vi "Overlay Results (Clamp).vi"(4 "Min / Max":bool, 5 "Setup":T3, 6 "Perpendicular Lines":T2(array[cluster]) {"?"."Y" format="%.2f"; "?"."X" format="%.2f"; "?"."Y" format="%.2f"; "?"."X" format="%.2f"}, 7 "ROI Descriptor":T1 {"Contours"."Type" items=["No Selection", "Point", "Line", "Rectangle", "Oval", "Polygon", "Free", "Annulus", "Unused2", "Unused3", "Broken Line", "Free Hand Line", "Rotated Rectangle"]}, 8 "Search Lines":T2(array[cluster]) {"?"."Y" format="%.2f"; "?"."X" format="%.2f"; "?"."Y" format="%.2f"; "?"."X" format="%.2f"}, 9 "All Edges Found":cluster{"X":sgl, "Y":sgl}[](array[cluster])=[{"X"=27.450102, "Y"=144.0}, {"X"=70.80146, "Y"=144.0}, {"X"=114.11963, "Y"=144.0}, {"X"=158.60345, "Y"=144.0}, {"X"=202.3678, "Y"=144.0}, {"X"=246.04292, "Y"=144.0}, {"X"=291.42203, "Y"=144.0}, {"X"=336.54822, "Y"=144.0}, {"X"=379.2348, "Y"=144.0}, {"X"=425.02194, "Y"=144.0}, {"X"=467.72144, "Y"=144.0}, {"X"=26.88918, "Y"=210.0}, {"X"=70.6191, "Y"=210.0}, {"X"=115.31038, "Y"=210.0}, {"X"=159.03351, "Y"=210.0}, {"X"=202.2118, "Y"=210.0}, {"X"=247.37573, "Y"=210.0}, {"X"=292.001, "Y"=210.0}, {"X"=336.55954, "Y"=210.0}, {"X"=379.72208, "Y"=210.0}, {"X"=424.86005, "Y"=210.0}, {"X"=468.8485, "Y"=210.0}, {"X"=26.897532, "Y"=309.0}, {"X"=70.88008, "Y"=309.0}, {"X"=114.93419, "Y"=309.0}, {"X"=159.13483, "Y"=309.0}, {"X"=203.12064, "Y"=309.0}, {"X"=247.9202, "Y"=309.0}, {"X"=291.07425, "Y"=309.0}, {"X"=335.25354, "Y"=309.0}, {"X"=378.88284, "Y"=309.0}, {"X"=424.06085, "Y"=309.0}, {"X"=469.80658, "Y"=309.0}] {"Y" format="%.2f"; "X" format="%.2f"}, 10 "Measurement Edges":cluster{"X":sgl, "Y":sgl}[](array[cluster])=[{"X"=27.450102, "Y"=144.0}, {"X"=70.80146, "Y"=144.0}, {"X"=114.11963, "Y"=144.0}, {"X"=158.60345, "Y"=144.0}, {"X"=202.3678, "Y"=144.0}, {"X"=246.04292, "Y"=144.0}, {"X"=291.42203, "Y"=144.0}, {"X"=336.54822, "Y"=144.0}, {"X"=379.2348, "Y"=144.0}, {"X"=425.02194, "Y"=144.0}, {"X"=467.72144, "Y"=144.0}, {"X"=26.88918, "Y"=210.0}, {"X"=70.6191, "Y"=210.0}, {"X"=115.31038, "Y"=210.0}, {"X"=159.03351, "Y"=210.0}, {"X"=202.2118, "Y"=210.0}, {"X"=247.37573, "Y"=210.0}, {"X"=292.001, "Y"=210.0}, {"X"=336.55954, "Y"=210.0}, {"X"=379.72208, "Y"=210.0}, {"X"=424.86005, "Y"=210.0}, {"X"=468.8485, "Y"=210.0}, {"X"=26.897532, "Y"=309.0}, {"X"=70.88008, "Y"=309.0}, {"X"=114.93419, "Y"=309.0}, {"X"=159.13483, "Y"=309.0}, {"X"=203.12064, "Y"=309.0}, {"X"=247.9202, "Y"=309.0}, {"X"=291.07425, "Y"=309.0}, {"X"=335.25354, "Y"=309.0}, {"X"=378.88284, "Y"=309.0}, {"X"=424.06085, "Y"=309.0}, {"X"=469.80658, "Y"=309.0}] {"Y" format="%.2f"; "X" format="%.2f"}, 11 "Image In":T4) -> (3 "Image Out":T4)   [LabVIEW 2020]
uses:
  IMAQ Image.ctl
panel:
  in  "Result Color":u32(colorbox)=16711680
  in  "Edge Locations Color":u32(colorbox)=16776960
  in  "Search Lines Color":u32(colorbox)=26367
  in  "Search Area Color":u32(colorbox)=65280
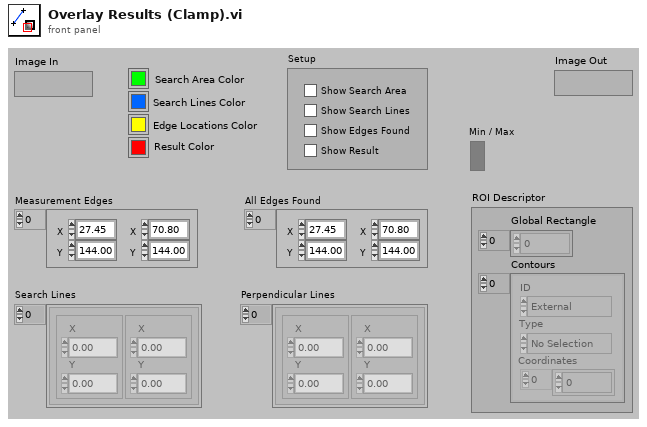
[diagram p1: front panel]
types:
  T1 = cluster{"Global Rectangle":i32[], "Contours":cluster{"ID":enum32{"External", "Internal"}, "Type":u32, "Coordinates":i32[]}[]}
  T2 = cluster{cluster{"X":sgl, "Y":sgl}, cluster{"X":sgl, "Y":sgl}}[]
  T3 = cluster{"Show Search Area":bool, "Show Search Lines":bool, "Show Edges Found":bool, "Show Result":bool}
  T4 = typedef "IMAQ Image.ctl" = refnum<image>
  T5 = cluster{"[0]":sgl, "[1]":sgl, "[2]":sgl, "[3]":sgl}
  T6 = cluster{"Perpendicular Lines[0]":cluster{cluster{"X":sgl, "Y":sgl}, cluster{"X":sgl, "Y":sgl}}, "Perpendicular Lines[1]":cluster{cluster{"X":sgl, "Y":sgl}, cluster{"X":sgl, "Y":sgl}}}
  T7 = cluster{cluster{"X":sgl, "Y":sgl}, cluster{"X":sgl, "Y":sgl}}
  T8 = cluster{cluster{"X":dbl, "Y":dbl}, cluster{"X":dbl, "Y":dbl}}
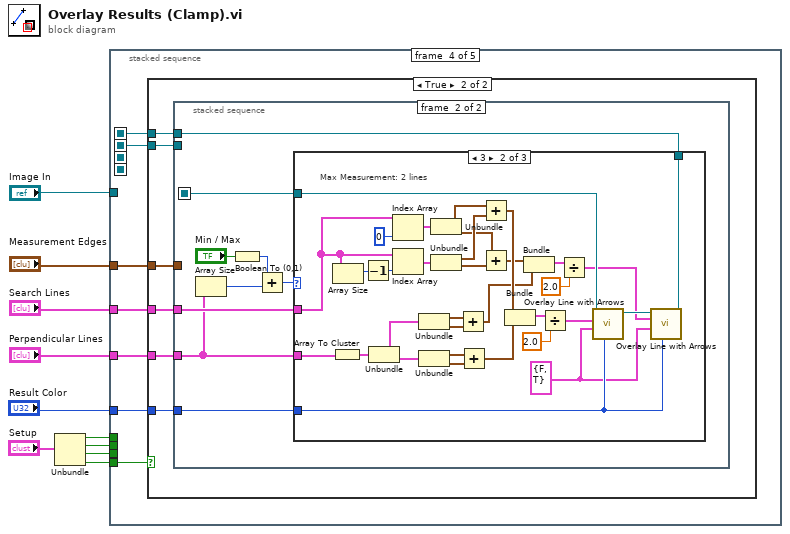
[diagram p0: block diagram]
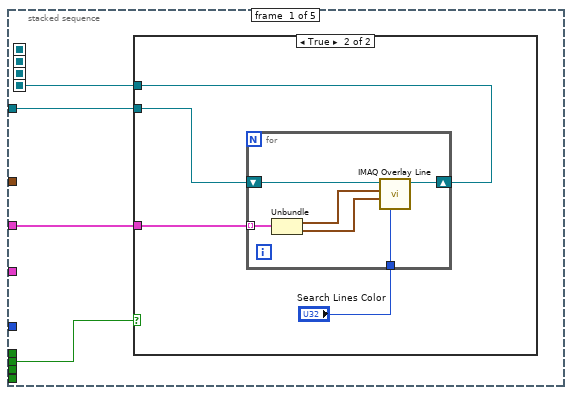
[diagram p2: hidden frame]
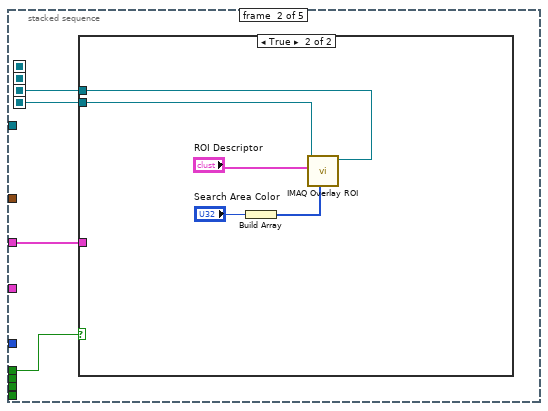
[diagram p4: hidden frame]
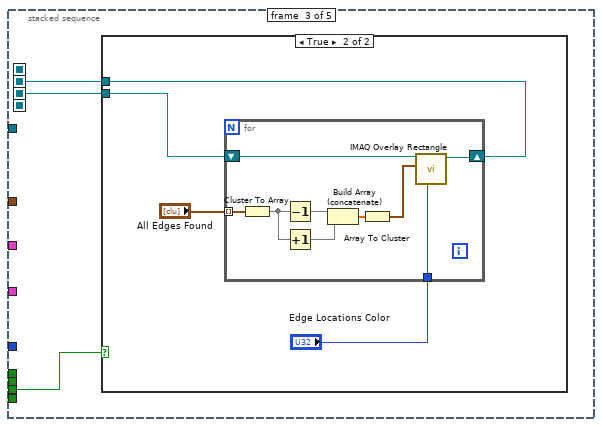
[diagram p6: hidden frame]
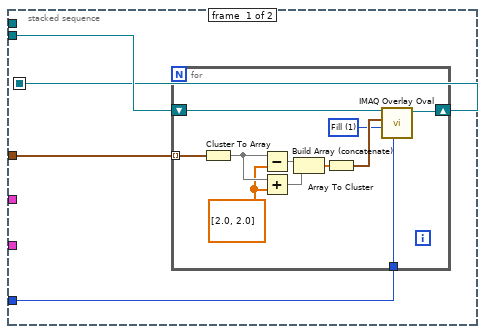
[diagram p9: hidden frame]
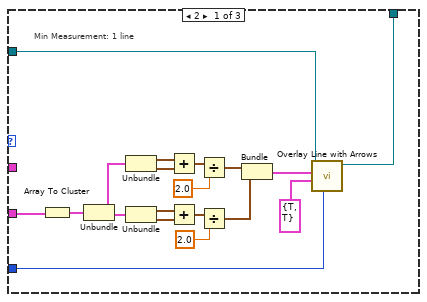
[diagram p10: hidden frame]
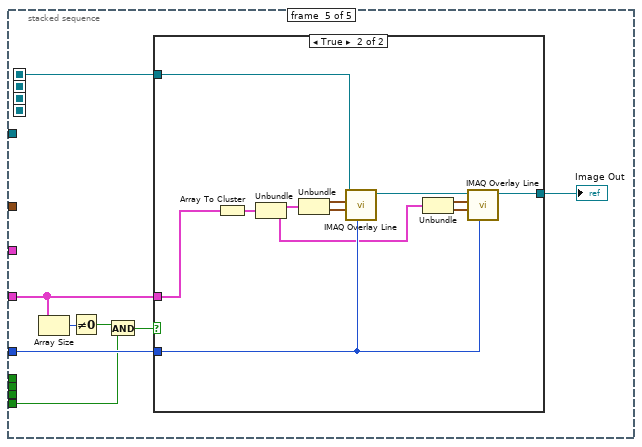
[diagram p12: hidden frame]
diagram:
  n1 = Unbundle("Setup") -> ("Show Search Area"=w4:bool, "Show Search Lines"=w5:bool, "Show Edges Found"=w3:bool, "Show Result"=w2:bool)
  n2 = stacked-sequence {
    seq-local: [_ _ w38 _ _] -> [_ _ _ w59 _]
    seq-local: [w13 _ _ _ _] -> [_ w28 _ _ _]
    seq-local: [_ w29 _ _ _] -> [_ _ w37 _ _]
    seq-local: [_ _ _ w58 _] -> [_ _ _ _ w149]
    tunnel: "Image In" -> [w14 _ _ _ _]
    tunnel: "Search Lines" -> [w12 w27 _ w53 _]
    tunnel: "Result Color" -> [_ _ _ w57 w150]
    tunnel: "Measurement Edges" -> [_ _ _ w56 _]
    tunnel: w5 -> [w11 _ _ _ _]
    tunnel: w4 -> [_ w26 _ _ _]
    tunnel: w3 -> [_ _ w36 _ _]
    tunnel: w2 -> [_ _ _ w55 w145]
    tunnel: "Perpendicular Lines" -> [_ _ _ w54 w148]
    frame #0 {
      n3 = case shown="True" w11 {
        tunnel: w14 -> [w15 w19]
        tunnel: [w15 w17] -> w13
        tunnel: w12 -> [_ w16]
        frame False {
        }
        frame True {
          n4 = for {
            shift-right: [w25] -> w17
            shift-left: w19 -> [w21]
            tunnel: "Search Lines Color" -> [w24]
            tunnel: w16 -> [w23] mode=indexing
            n5 = Unbundle(w23) -> (w20:cluster{"X":sgl, "Y":sgl}, w22:cluster{"X":sgl, "Y":sgl})
            n6 = call "IMAQ Overlay Line"("Color"=w24, "End Point"=w22, "Start Point"=w20, "Image"=w21) -> ("Image Out"=w25:T4)  [unwired: 2 in, 5 out]
          }
        }
      }
    }
    frame #1 {
      n7 = case shown="True" w26 {
        tunnel: [w30 w33] -> w29
        tunnel: w28 -> [w30 w34]
        tunnel: w27 -> [_ _]
        frame False {
        }
        frame True {
          n8 = Build Array("Search Area Color") -> (w31:u32[])
          n9 = call "IMAQ Overlay ROI"("Colors (Green)"=w31, "ROI Descriptor"="ROI Descriptor", "Image"=w34) -> ("Image Out"=w33:T4)  [unwired: 3 in, 5 out]
        }
      }
    }
    frame #2 {
      n10 = case shown="True" w36 {
        tunnel: [w39 w43] -> w38
        tunnel: w37 -> [w39 w42]
        frame False {
        }
        frame True {
          n11 = for {
            shift-right: [w51] -> w43
            shift-left: w42 -> [w52]
            tunnel: "All Edges Found" -> [w50] mode=indexing
            tunnel: "Edge Locations Color" -> [w49]
            n12 = Cluster To Array(cluster=w50) -> (array=w45:sgl[])
            n13 = Decrement(x=w45) -> (x-1=w48:sgl[])
            n14 = Increment(x=w45) -> (x+1=w44:sgl[])
            n15 = Build Array (concatenate)(w48, w44) -> (w47:sgl[])
            n16 = Array To Cluster(array=w47) -> (cluster=w46:T5)
            n17 = call "IMAQ Overlay Rectangle"("Color"=w49, "Rectangle"=w46, "Image"=w52) -> ("Image Out"=w51:T4)  [unwired: 3 in, 5 out]
          }
        }
      }
    }
    frame #3 {
      n18 = case shown="True" w55 {
        tunnel: w59 -> [w60 w66]
        tunnel: [w60 w63] -> w58
        tunnel: w57 -> [_ w65]
        tunnel: w56 -> [_ w64]
        tunnel: w54 -> [_ w62]
        tunnel: w53 -> [_ w61]
        frame False {
        }
        frame True {
          n19 = stacked-sequence {
            seq-local: [w67 _] -> [_ w89]
            tunnel: w66 -> [w70 _]
            tunnel: w65 -> [w69 w90]
            tunnel: w64 -> [w68 _]
            tunnel: [_ w88] -> w63
            tunnel: w62 -> [_ w86]
            tunnel: w61 -> [_ w87]
            frame #0 {
              n20 = for {
                shift-right: [w80] -> w67
                shift-left: w70 -> [w81]
                tunnel: w68 -> [w79] mode=indexing
                tunnel: w69 -> [w72]
                w71 = u32 1 items=["Frame", "Fill"] ("Drawing Mode (Frame)")
                w73 = sgl[] [2.0, 2.0] ("y")
                n21 = Cluster To Array(cluster=w79) -> (array=w78:sgl[])
                n22 = Subtract(x=w78, y=w73) -> (x-y=w77:sgl[])
                n23 = Add(x=w78, y=w73) -> (x+y=w76:sgl[])
                n24 = Build Array (concatenate)(w77, w76) -> (w75:sgl[])
                n25 = Array To Cluster(array=w75) -> (cluster=w74:T5)
                n26 = call "IMAQ Overlay Oval"("Color"=w72, "Drawing Mode (Frame)"=w71, "Bounding Rectangle"=w74, "Image"=w81) -> ("Image Out"=w80:T4)  [unwired: 2 in, 5 out]
              }
            }
            frame #1 {
              n27 = Array Size(array=w86) -> (size(s)=w84:i32)
              n28 = Boolean To (0,1)(Boolean="Min / Max") -> (0, 1=w83:i16)
              n29 = Add(x=w83, y=w84) -> (x+y=w82:i32)
              n30 = case shown="3" w82 {
                tunnel: w90 -> [w109 w126 _]
                tunnel: w89 -> [w108 w142 w143]
                tunnel: [w107 w124 w143] -> w88
                tunnel: w86 -> [w91 w134 _]
                tunnel: w87 -> [_ w128 _]
                frame 2 {
                  # "Min Measurement: 1 line"
                  n31 = Array To Cluster(array=w91) -> (cluster=w104:T6)
                  n32 = Unbundle(w104) -> ("Perpendicular Lines[0]"=w103:T7, "Perpendicular Lines[1]"=w94:T7)
                  n33 = Unbundle(w103) -> (w102:cluster{"X":sgl, "Y":sgl}, w101:cluster{"X":sgl, "Y":sgl})
                  n34 = Unbundle(w94) -> (w95:cluster{"X":sgl, "Y":sgl}, w96:cluster{"X":sgl, "Y":sgl})
                  n35 = Add(x=w102, y=w101) -> (x+y=w100:cluster{"X":sgl, "Y":sgl})
                  n36 = Add(x=w95, y=w96) -> (x+y=w97:cluster{"X":sgl, "Y":sgl})
                  n37 = Divide(x=w100, y=2.0) -> (x/y=w93:cluster{"X":dbl, "Y":dbl})
                  n38 = Divide(x=w97, y=2.0) -> (x/y=w92:cluster{"X":dbl, "Y":dbl})
                  n39 = Bundle(w93, w92) -> (w105:T8)  [unwired: 1 out]
                  n40 = call "Overlay Line with Arrows.vi"("Color"=w109, "Arrows"=cluster{"Start point":bool, "End point":bool} {"Start point"=TRUE, "End point"=TRUE}, "Line Coordinates"=w105, "Image In"=w108) -> ("Image Out"=w107:T4)  [unwired: 2 in, 5 out]
                }
                frame 3 {
                  w125 = cluster{"Start point":bool, "End point":bool} {"Start point"=FALSE, "End point"=TRUE} ("Arrows")
                  # "Max Measurement: 2 lines"
                  n41 = Array To Cluster(array=w134) -> (cluster=w141:T6)
                  n42 = Array Size(array=w128) -> (size(s)=w133:i32)
                  n43 = Decrement(x=w133) -> (x-1=w132:i32)
                  n44 = Unbundle(w141) -> ("Perpendicular Lines[0]"=w140:T7, "Perpendicular Lines[1]"=w135:T7)
                  n45 = Index Array(array=w128, index=0 ("Index")) -> (element=w131:T7)
                  n46 = Index Array(array=w128, index=w132) -> (element=w130:T7)
                  n47 = Unbundle(w140) -> (w139:cluster{"X":sgl, "Y":sgl}, w138:cluster{"X":sgl, "Y":sgl})
                  n48 = Unbundle(w135) -> (w136:cluster{"X":sgl, "Y":sgl}, w137:cluster{"X":sgl, "Y":sgl})
                  n49 = Unbundle(w131) -> (w123:cluster{"X":sgl, "Y":sgl}, w121:cluster{"X":sgl, "Y":sgl})
                  n50 = Unbundle(w130) -> (w122:cluster{"X":sgl, "Y":sgl}, w120:cluster{"X":sgl, "Y":sgl})
                  n51 = Add(x=w139, y=w138) -> (x+y=w117:cluster{"X":sgl, "Y":sgl})
                  n52 = Add(x=w136, y=w137) -> (x+y=w116:cluster{"X":sgl, "Y":sgl})
                  n53 = Add(x=w123, y=w122) -> (x+y=w119:cluster{"X":sgl, "Y":sgl})
                  n54 = Add(x=w121, y=w120) -> (x+y=w118:cluster{"X":sgl, "Y":sgl})
                  n55 = Bundle(w119, w116) -> (w115:T7)  [unwired: 1 out]
                  n56 = Bundle(w118, w117) -> (w113:T7)  [unwired: 1 out]
                  n57 = Divide(x=w115, y=2.0) -> (x/y=w114:T8)
                  n58 = Divide(x=w113, y=2.0) -> (x/y=w112:T8)
                  n59 = call "Overlay Line with Arrows.vi"("Color"=w126, "Arrows"=w125, "Line Coordinates"=w114, "Image In"=w142) -> ("Image Out"=w127:T4)  [unwired: 2 in, 5 out]
                  n60 = call "Overlay Line with Arrows.vi"("Color"=w126, "Arrows"=w125, "Line Coordinates"=w112, "Image In"=w127) -> ("Image Out"=w124:T4)  [unwired: 2 in, 5 out]
                }
                frame Default {
                  # "No perpendicular line: no arrow needed."
                }
              }
            }
          }
        }
      }
    }
    frame #4 {
      n61 = Array Size(array=w148) -> (size(s)=w147:i32)
      n62 = Not Equal To 0?(x=w147) -> (x != 0?=w146:bool)
      n63 = And(x=w146, y=w145) -> (x .and. y?=w144:bool)
      n64 = case shown="True" w144 {
        tunnel: [w152 w164] -> w151
        tunnel: w150 -> [_ w163]
        tunnel: w149 -> [w152 w156]
        tunnel: w148 -> [_ w157]
        frame False {
        }
        frame True {
          n65 = Array To Cluster(array=w157) -> (cluster=w162:T6)
          n66 = Unbundle(w162) -> ("Perpendicular Lines[0]"=w161:T7, "Perpendicular Lines[1]"=w160:T7)
          n67 = Unbundle(w161) -> (w153:cluster{"X":sgl, "Y":sgl}, w159:cluster{"X":sgl, "Y":sgl})
          n68 = call "IMAQ Overlay Line"("Color"=w163, "End Point"=w159, "Start Point"=w153, "Image"=w156) -> ("Image Out"=w155:T4)  [unwired: 2 in, 5 out]
          n69 = Unbundle(w160) -> (w154:cluster{"X":sgl, "Y":sgl}, w158:cluster{"X":sgl, "Y":sgl})
          n70 = call "IMAQ Overlay Line"("Color"=w163, "End Point"=w158, "Start Point"=w154, "Image"=w155) -> ("Image Out"=w164:T4)  [unwired: 2 in, 5 out]
        }
      }
      "Image Out" <- w151
    }
  }
